vi "MakeExample.vi"(8 "error in (no error)":errorcluster, 9 "TriggerRefractoryPeriod (Frames)":i32, 10 "StimulusObject Parameters":variant, 11 "StimulateReversingWorms in":refnum<class "StimulateReversingWorms.lvclass">) -> (0 "error out":errorcluster, 3 "StimulateReversingWorms out":refnum<class "StimulateReversingWorms.lvclass">)   [LabVIEW 2019, in "StimulateReversingWorms.lvclass"]
uses:
  StimulateReversingWorms.lvclass
  StimulateReversingWormsInputCluster.ctl
  StimulateReversingWorms.lvclass/StimulateReversingWorms.ctl
  ParametersGlobal.vi
  StimulusObject.lvclass
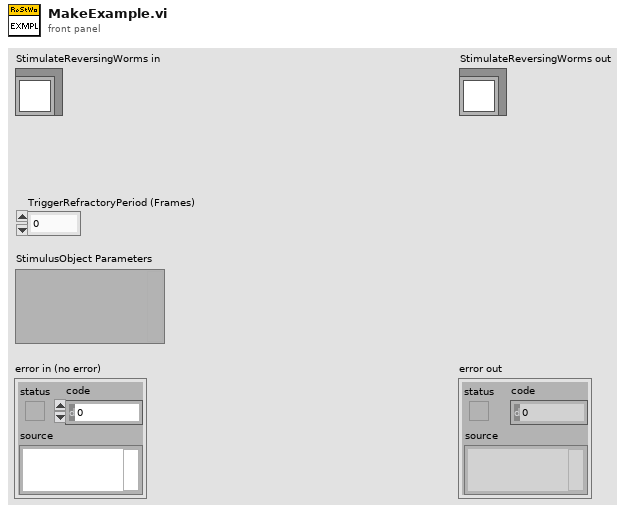
[diagram p1: front panel]
types:
  T1 = typedef "StimulateReversingWorms.lvclass/StimulateReversingWormsInputCluster.ctl" = cluster{"Constant Intensity (uW/mm^2, negative is blue)":sgl, "dot radius (mm)":sgl, "Intensities (uW/mm^2, negative is blue)":sgl[], "Durations (s)":sgl[], "Inter trigger interval (s)":dbl, "Wait time after reversal is detected (s)":dbl}
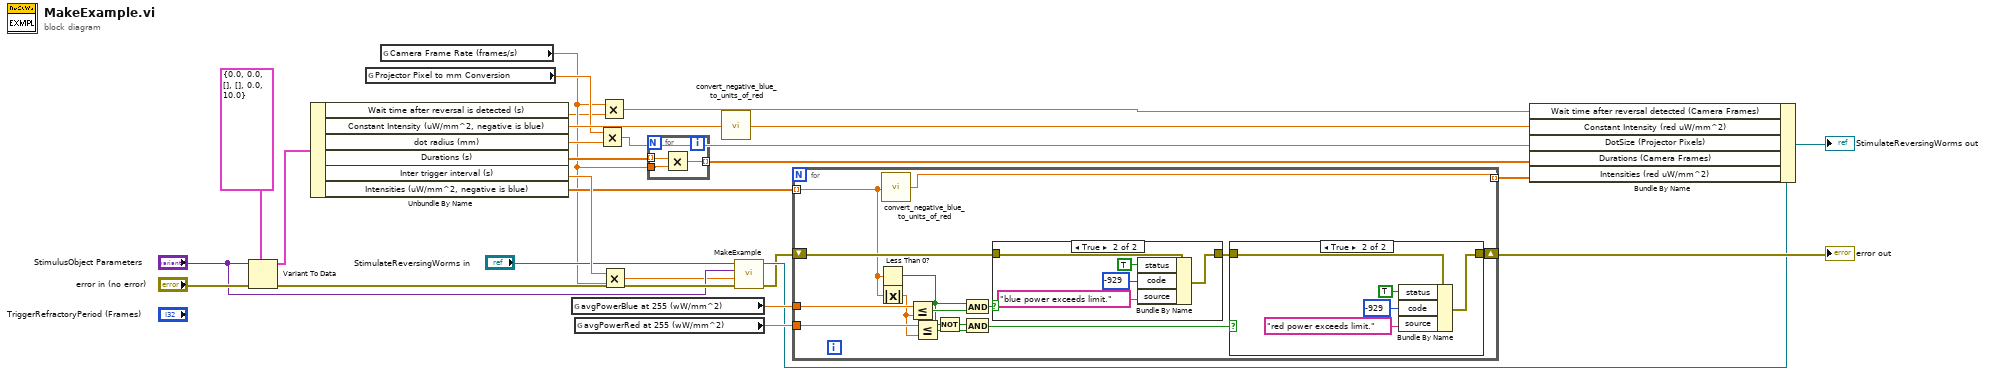
[diagram p0: block diagram]
diagram:
  n1 = Variant To Data(error in="error in (no error)", type=T1 {"Constant Intensity (uW/mm^2, negative is blue)"=0.0, "dot radius (mm)"=0.0, "Intensities (uW/mm^2, negative is blue)"=[], "Durations (s)"=[], "Inter trigger interval (s)"=0.0, "Wait time after reversal is detected (s)"=10.0} ("StimulateReversingWormsInputCluster"), Variant="StimulusObject Parameters") -> (data=w25:T1, error out=w9:errorcluster)
  n2 = Unbundle By Name(w25) -> ("Wait time after reversal is detected (s)"=w2:dbl, "Constant Intensity (uW/mm^2, negative is blue)"=w23:sgl, "dot radius (mm)"=w21:sgl, "Durations (s)"=w18:sgl[], "Inter trigger interval (s)"=w24:dbl, "Intensities (uW/mm^2, negative is blue)"=w16:sgl[])
  n3 = global read "ParametersGlobal.vi" "Projector Pixel to mm Conversion"() -> (w20:sgl)
  n4 = global read "ParametersGlobal.vi" "Camera Frame Rate (frames/s)"() -> (w3:sgl)
  n5 = global read "ParametersGlobal.vi" "avgPowerBlue at 255 (wW/mm^2)"() -> (w15:sgl)
  n6 = global read "ParametersGlobal.vi" "avgPowerRed at 255 (wW/mm^2)"() -> (w14:sgl)
  n7 = Multiply(x=w20, y=w21) -> (x*y=w19:sgl)
  n8 = Multiply(x=w3, y=w2) -> (x*y=w1:dbl)
  n9 = Multiply(x=w24, y=w3) -> (x*y=w7:dbl)
  n10 = for {
    tunnel: w18 -> [w29] mode=indexing
    tunnel: w3 -> [w28]
    tunnel: [w27] -> w17 mode=indexing
    n11 = Multiply(x=w29, y=w28) -> (x*y=w27:sgl)
  }
  n12 = call "convert_negative_blue_to_units_of_red.vi"("Intensity in units of red (positive) and blue (negative)"=w23) -> ("Intensity in units of red (positive and negative)"=w22:sgl)
  n13 = call-parent "MakeExample.vi"("error in (no error)"=w9, "TriggerRefractoryPeriod (Frames)"=w7, "StimulusObject Parameters"="StimulusObject Parameters", "StimulusObject in"="StimulateReversingWorms in") -> ("error out"=w4:errorcluster, "StimulusObject out"=w5:refnum<class "StimulateReversingWorms.lvclass">)  [unwired: 6 in]
  n14 = for {
    tunnel: w16 -> [w37] mode=indexing
    shift-right: [w41] -> w10
    shift-left: w4 -> [w42]
    tunnel: w15 -> [w40]
    tunnel: w14 -> [w39]
    tunnel: [w38] -> w13 mode=indexing
    n15 = Less Than 0?(x=w37) -> (x < 0?=w30:bool)
    n16 = Absolute Value(x=w37) -> (abs(x)=w36:sgl)
    n17 = call "convert_negative_blue_to_units_of_red.vi"("Intensity in units of red (positive) and blue (negative)"=w37) -> ("Intensity in units of red (positive and negative)"=w38:sgl)
    n18 = Less Or Equal?(x=w40, y=w36) -> (x <= y?=w35:bool)
    n19 = Less Or Equal?(x=w39, y=w36) -> (x <= y?=w32:bool)
    n20 = Not(x=w30) -> (.not. x?=w31:bool)
    n21 = And(x=w30, y=w35) -> (x .and. y?=w34:bool)
    n22 = And(x=w31, y=w32) -> (x .and. y?=w33:bool)
    n23 = case shown="True" w34 {
      tunnel: w42 -> [w50 w55]
      tunnel: [w50 w54] -> w43
      frame False {
      }
      frame True {
        n24 = Bundle By Name(cluster=w55, "status"=TRUE, "code"=-929, "source"="blue power exceeds limit.") -> (w54:errorcluster)
      }
    }
    n25 = case shown="True" w33 {
      tunnel: w43 -> [w44 w49]
      tunnel: [w44 w48] -> w41
      frame False {
      }
      frame True {
        n26 = Bundle By Name(cluster=w49, "status"=TRUE, "code"=-929, "source"="red power exceeds limit.") -> (w48:errorcluster)
      }
    }
  }
  "error out" <- w10
  n27 = Bundle By Name(cluster=w5, "Wait time after reversal detected (Camera Frames)"=w1, "Constant Intensity (red uW/mm^2)"=w22, "DotSize (Projector Pixels)"=w19, "Durations (Camera Frames)"=w17, "Intensities (red uW/mm^2)"=w13) -> (→"StimulateReversingWorms out":refnum<class "StimulateReversingWorms.lvclass">)
